vi "Timer.vi"(7 "Timer Command":T1=enum."Start", 8 "Error In":errorcluster, 9 "name qualifier (empty if unwired)":string, 10 "VI name (Optional)":string, 11 "Set Time IN (s)":dbl) -> (0 "Error Out":errorcluster, 1 "Remaining Time (s)":dbl, 2 "Elapsed Time (s)":dbl, 3 "Complete?":bool, 4 "Set Time OUT (s)":dbl, 5 "Calling VI OUT":string)   [LabVIEW 2017]
doc: "SciScan 1.2 160622\nThis FGV implements a timer.\nFunctionality is a follows:\n1. START the timer first (using the command enum and specifying the timing duration.\n2. Calling the VI with 'RUN' returns the elapsed time, remaining time and indication weather complete\n3. A PAUSE functionality is also provided which allows you to suspend the timing till RUN is called again"
uses:
  Timer Commands.ctl
panel:
  out "date/time string":string
  out "Boolean":bool
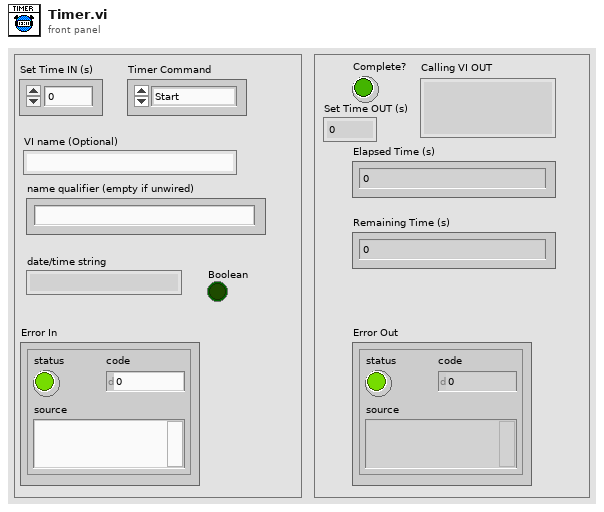
[diagram p1: front panel]
types:
  T1 = typedef "Timer Commands.ctl" = enum16{"Clear All", "Start", "Pause", "Check Time"}
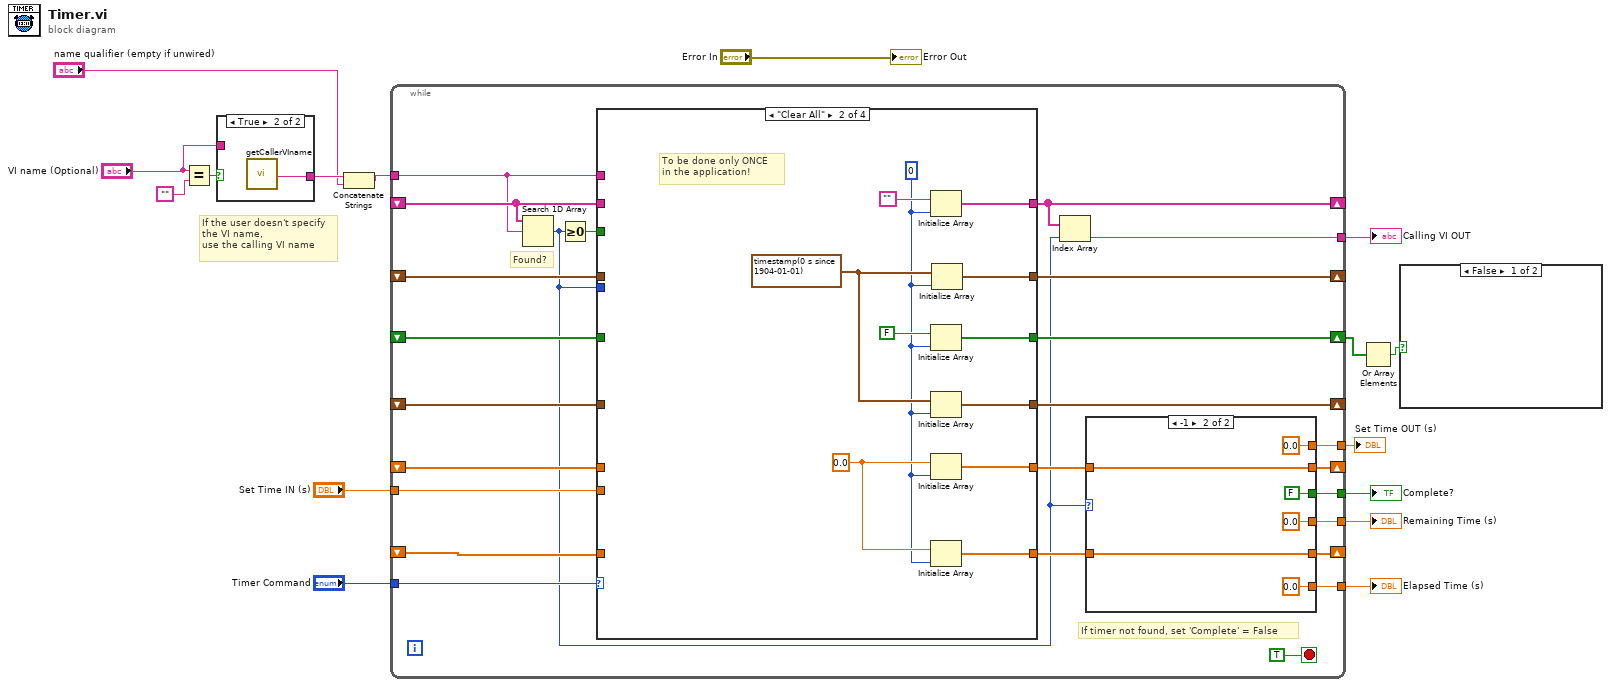
[diagram p0: block diagram]
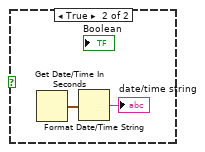
[diagram p2: hidden frame]
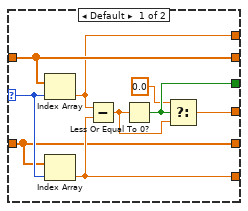
[diagram p4: hidden frame]
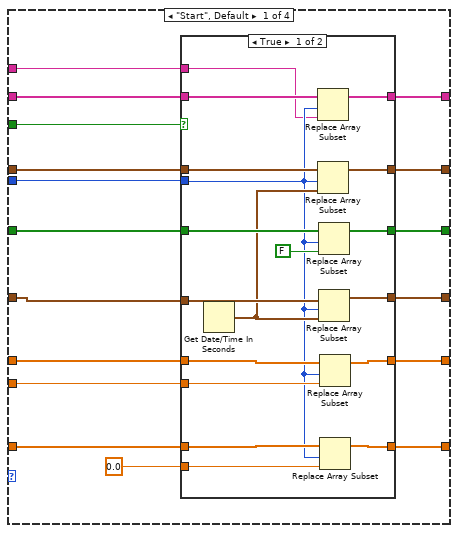
[diagram p5: hidden frame]
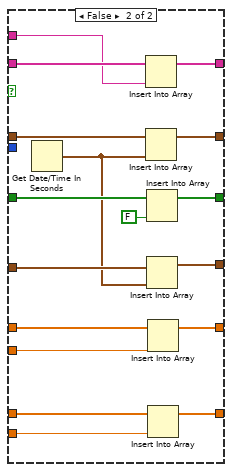
[diagram p6: hidden frame]
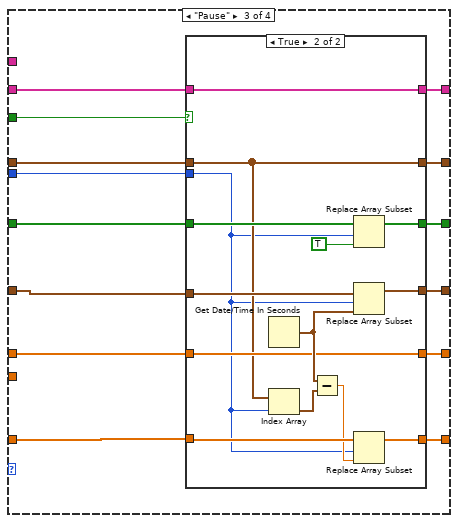
[diagram p7: hidden frame]
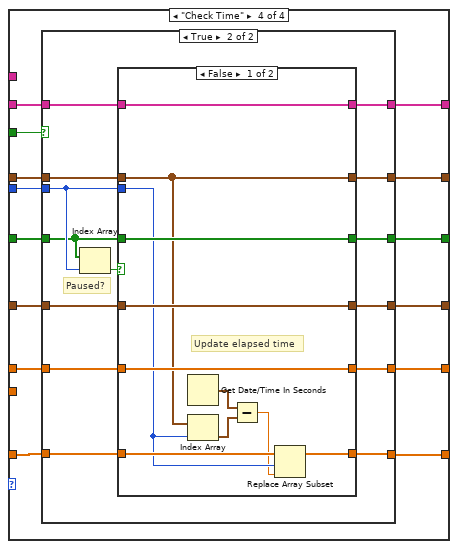
[diagram p9: hidden frame]
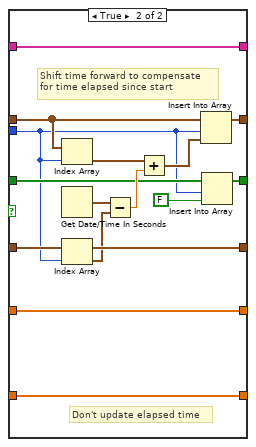
[diagram p11: hidden frame]
diagram:
  # "If the user doesn't specify\nthe VI name,\nuse the calling VI name"
  n1 = Equal?(x="VI name (Optional)", y="") -> (x = y?=w8:bool)
  n2 = case shown="True" w8 {
    tunnel: [w17 w18] -> w7
    tunnel: "VI name (Optional)" -> [w17 _]
    frame False {
    }
    frame True {
      n3 = call "getCallerVIname.vi"() -> ("VI name"=w18:string)  [unwired: 19 in]
    }
  }
  n4 = Concatenate Strings(w7, "name qualifier (empty if unwired)") -> (w5:string)
  n5 = while {
    tunnel: "Timer Command" -> [w42]
    shift-right: [w21] -> _
    shift-left: _ -> [w37]
    shift-right: [w41] -> _
    shift-left: _ -> [w40]
    shift-right: [w39] -> w4
    shift-left: _ -> [w38]
    shift-right: [w36] -> _
    shift-left: _ -> [w35]
    shift-right: [w20] -> _
    shift-left: _ -> [w34]
    tunnel: [w33] -> w12
    tunnel: [w27] -> w11
    shift-right: [w25] -> _
    shift-left: _ -> [w31]
    tunnel: "Set Time IN (s)" -> [w32]
    tunnel: [w26] -> w13
    tunnel: [w24] -> w10
    tunnel: w5 -> [w23]
    tunnel: [w19] -> w1
    stop <- TRUE stop-if-true
    # "If timer not found, set 'Complete' = False"
    # "Found?"
    n6 = Search 1D Array(1D array=w31, element=w23) -> (index of element=w22:i32)  [unwired: 1 in]
    n7 = Greater Or Equal To 0?(x=w22) -> (x >= 0?=w30:bool)
    n8 = case shown="\"Clear All\"" w42 {
      tunnel: [w67 w114 w125 w161] -> w29
      tunnel: [w74 w119 w131 w165] -> w41
      tunnel: w40 -> [w75 _ w133 w168]
      tunnel: [w71 w112 w135 w159] -> w39
      tunnel: w38 -> [w73 _ w128 w169]
      tunnel: w37 -> [w66 _ w126 w166]
      tunnel: [w69 w113 w134 w162] -> w36
      tunnel: w35 -> [w70 _ w127 w167]
      tunnel: [w63 w111 w132 w164] -> w28
      tunnel: w34 -> [w65 _ w124 w163]
      tunnel: [w72 w120 w129 w160] -> w25
      tunnel: w31 -> [w59 _ w130 w157]
      tunnel: w32 -> [w68 _ _ _]
      tunnel: w30 -> [w61 _ w123 w158]
      tunnel: w22 -> [w62 _ w122 w156]
      tunnel: w23 -> [w60 _ _ _]
      frame "Start", Default {
        n9 = case shown="True" w61 {
          tunnel: w59 -> [w93 w110]
          tunnel: w62 -> [w79 _]
          tunnel: w75 -> [w92 w109]
          tunnel: [w91 w108] -> w74
          tunnel: w73 -> [w90 w107]
          tunnel: [w88 w105] -> w72
          tunnel: [w87 w104] -> w71
          tunnel: w70 -> [w86 w103]
          tunnel: [w84 w101] -> w69
          tunnel: w68 -> [w83 w100]
          tunnel: [w82 w99] -> w67
          tunnel: w66 -> [w81 w98]
          tunnel: w65 -> [w80 w97]
          tunnel: 0.0 -> [w78 w96]
          tunnel: [w77 w95] -> w63
          tunnel: w60 -> [w76 w94]
          frame True {
            n10 = Get Date/Time In Seconds() -> (seconds since 1Jan1904=w85:timestamp)
            n11 = Replace Array Subset(array=w93, new element=w76, index=w79) -> (w88:string[])
            n12 = Replace Array Subset(array=w92, new element=w85, index=w79) -> (w91:timestamp[])
            n13 = Replace Array Subset(array=w90, new element=FALSE, index=w79) -> (w87:bool[])
            n14 = Replace Array Subset(array=w86, new element=w85, index=w79) -> (w84:timestamp[])
            n15 = Replace Array Subset(array=w81, new element=w83, index=w79) -> (w82:dbl[])
            n16 = Replace Array Subset(array=w80, new element=w78, index=w79) -> (w77:dbl[])
          }
          frame False {
            n17 = Get Date/Time In Seconds() -> (seconds since 1Jan1904=w102:timestamp)
            n18 = Insert Into Array(array=w110, new element=w94) -> (w105:string[])  [unwired: 1 in]
            n19 = Insert Into Array(array=w109, new element=w102) -> (w108:timestamp[])  [unwired: 1 in]
            n20 = Insert Into Array(array=w107, new element=FALSE) -> (w104:bool[])  [unwired: 1 in]
            n21 = Insert Into Array(array=w103, new element=w102) -> (w101:timestamp[])  [unwired: 1 in]
            n22 = Insert Into Array(array=w98, new element=w100) -> (w99:dbl[])  [unwired: 1 in]
            n23 = Insert Into Array(array=w97, new element=w96) -> (w95:dbl[])  [unwired: 1 in]
          }
        }
      }
      frame "Clear All" {
        w116 = 0.0 ("Set Time (s)")
        w117 = timestamp(0 s since 1904-01-01) ("current time")
        w115 = 0 ("dimension size")
        # "To be done only ONCE\nin the application!"
        n24 = Initialize Array("", w115) -> (w120:string[])
        n25 = Initialize Array(FALSE, w115) -> (w112:bool[])
        n26 = Initialize Array(w117, w115) -> (w113:timestamp[])
        n27 = Initialize Array(w116, w115) -> (w114:dbl[])
        n28 = Initialize Array(w116, w115) -> (w111:dbl[])
        n29 = Initialize Array(w117, w115) -> (w119:timestamp[])
      }
      frame "Pause" {
        n30 = case shown="True" w123 {
          tunnel: [w139 w154] -> w135
          tunnel: [w138 w148] -> w134
          tunnel: w133 -> [w140 w147]
          tunnel: [w136 w142] -> w132
          tunnel: [w140 w147] -> w131
          tunnel: [w141 w155] -> w129
          tunnel: w130 -> [w141 w155]
          tunnel: w128 -> [w139 w153]
          tunnel: w122 -> [_ w143]
          tunnel: w127 -> [w138 w151]
          tunnel: w126 -> [w137 w149]
          tunnel: [w137 w149] -> w125
          tunnel: w124 -> [w136 w145]
          frame False {
            # "Caller not found!\n~~ Do Nothing ~~"
          }
          frame True {
            n31 = Get Date/Time In Seconds() -> (seconds since 1Jan1904=w150:timestamp)
            n32 = Index Array(array=w147, index=w143) -> (element=w146:timestamp)
            n33 = Subtract(x=w150, y=w146) -> (x-y=w144:dbl)
            n34 = Replace Array Subset(array=w153, new element=TRUE, index=w143) -> (w154:bool[])
            n35 = Replace Array Subset(array=w151, new element=w150, index=w143) -> (w148:timestamp[])
            n36 = Replace Array Subset(array=w145, new element=w144, index=w143) -> (w142:dbl[])
          }
        }
      }
      frame "Check Time" {
        n37 = case shown="True" w158 {
          tunnel: w169 -> [w173 w177]
          tunnel: w168 -> [w174 w189]
          tunnel: w167 -> [w172 w188]
          tunnel: w166 -> [w171 w187]
          tunnel: [w174 w186] -> w165
          tunnel: [w170 w185] -> w164
          tunnel: w163 -> [w170 w184]
          tunnel: [w172 w183] -> w162
          tunnel: [w171 w182] -> w161
          tunnel: w157 -> [w175 w181]
          tunnel: [w175 w180] -> w160
          tunnel: [w173 w176] -> w159
          tunnel: w156 -> [_ w179]
          frame False {
          }
          frame True {
            # "Paused?"
            n38 = Index Array(array=w177, index=w179) -> (element=w178:bool)
            n39 = case shown="False" w178 {
              tunnel: w189 -> [w195 w207]
              tunnel: w188 -> [w198 w210]
              tunnel: w187 -> [w199 w214]
              tunnel: [w195 w205] -> w186
              tunnel: [w190 w215] -> w185
              tunnel: w184 -> [w193 w215]
              tunnel: [w198 w210] -> w183
              tunnel: [w199 w214] -> w182
              tunnel: w181 -> [w196 w208]
              tunnel: w179 -> [w192 w203]
              tunnel: [w196 w208] -> w180
              tunnel: w177 -> [w197 w204]
              tunnel: [w197 w201] -> w176
              frame False {
                # "Update elapsed time"
                n40 = Get Date/Time In Seconds() -> (seconds since 1Jan1904=w200:timestamp)
                n41 = Index Array(array=w195, index=w192) -> (element=w194:timestamp)
                n42 = Subtract(x=w200, y=w194) -> (x-y=w191:dbl)
                n43 = Replace Array Subset(array=w193, new element=w191, index=w192) -> (w190:dbl[])
              }
              frame True {
                # "Don't update elapsed time"
                # "Shift time forward to compensate\nfor time elapsed since start"
                n44 = Index Array(array=w207, index=w203) -> (element=w211:timestamp)
                n45 = Get Date/Time In Seconds() -> (seconds since 1Jan1904=w213:timestamp)
                n46 = Index Array(array=w210, index=w203) -> (element=w209:timestamp)
                n47 = Subtract(x=w213, y=w209) -> (x-y=w212:dbl)
                n48 = Add(x=w211, y=w212) -> (x+y=w206:timestamp)
                n49 = Insert Into Array(array=w207, index=w203, new element=w206) -> (w205:timestamp[])
                n50 = Insert Into Array(array=w204, index=w203, new element=FALSE) -> (w201:bool[])
              }
            }
          }
        }
      }
    }
    n51 = Index Array(array=w25, index=w22) -> (element=w24:string)
    n52 = case shown="-1" w22 {
      selector: w22 -> [w47 _]
      tunnel: [w52 0.0 ("f")] -> w33
      tunnel: w29 -> [w46 w58]
      tunnel: w28 -> [w45 w57]
      tunnel: [w51 FALSE] -> w27
      tunnel: [w50 0.0 ("Set Time (s)")] -> w26
      tunnel: [w46 w58] -> w21
      tunnel: [w45 w57] -> w20
      tunnel: [w44 0.0 ("Set Time (s)")] -> w19
      frame Default {
        n53 = Index Array(array=w46, index=w47) -> (element=w44:dbl)
        n54 = Index Array(array=w45, index=w47) -> (element=w50:dbl)
        n55 = Subtract(x=w44, y=w50) -> (x-y=w48:dbl)
        n56 = Less Or Equal To 0?(x=w48) -> (x <= 0?=w51:bool)
        n57 = Select(t=0.0 ("f"), s=w51, f=w48) -> (s? t:f=w52:dbl)
      }
      frame -1 {
      }
    }
  }
  "Complete?" <- w11
  "Remaining Time (s)" <- w12
  "Elapsed Time (s)" <- w13
  "Calling VI OUT" <- w10
  "Set Time OUT (s)" <- w1
  n58 = Or Array Elements(Boolean array=w4) -> (logical OR=w3:bool)
  n59 = case shown="False" w3 {
    frame False {
    }
    frame True {
      n60 = Get Date/Time In Seconds() -> (seconds since 1Jan1904=w217:timestamp)
      n61 = Format Date/Time String(seconds (now)=w217) -> (date/time string=→"date/time string":string)  [unwired: 2 in]
    }
  }
  "Error Out" <- "Error In"
